vi "NIPKG to SBOM Component.vi"(8 "error in (no error)":errorcluster, 11 "nipkg package attributes":T1={"Package Name"="", "Display name"="", "Version"="", "Display version"="", "Synopsis"="", "Description"="", "Maintainer"="", "Maintainer email address"="", "Category"="", "Homepage"="", "Release notes"="", "Depends"=[], "Recommends"=[], "Suggests"=[], "Conflicts"=[], "Provides"=[], "Replaces"=[], "Supplements"=[], "Enhances"=[], "Product"=FALSE, "User visible"=FALSE, "Installed size (KB)"=0, "Package filesize (bytes)"=0, "Architecture"="", "Agent"="file", "MD5Checksum"=""}) -> (0 "error out":errorcluster, 3 "Component out":refnum<class "CycloneDX Component.lvclass">)   [LabVIEW 2017, in "NIPKG SBOM Support.lvlib"]
doc: "Converts NIPKG information to a CycloneDX SBOM component."
uses:
  NIPKG SBOM Support.lvlib
  <vilib>/National Instruments/NIPM API (Beta)/_support/package attributes.ctl
  CycloneDX/CycloneDX Component/CycloneDX Component.lvclass
  C:/LabVIEW Working Directory/labview-cyclonedx-sbom/Source/CycloneDX/CycloneDX JSON/CycloneDX JSON.lvclass
  CycloneDX/CycloneDX JSON/CycloneDX Types.ctl
  CycloneDX/CycloneDX JSON/CycloneDX JSON.lvclass
  <vilib>/National Instruments/NIPM API (Beta)/NIPM_API.lvlib
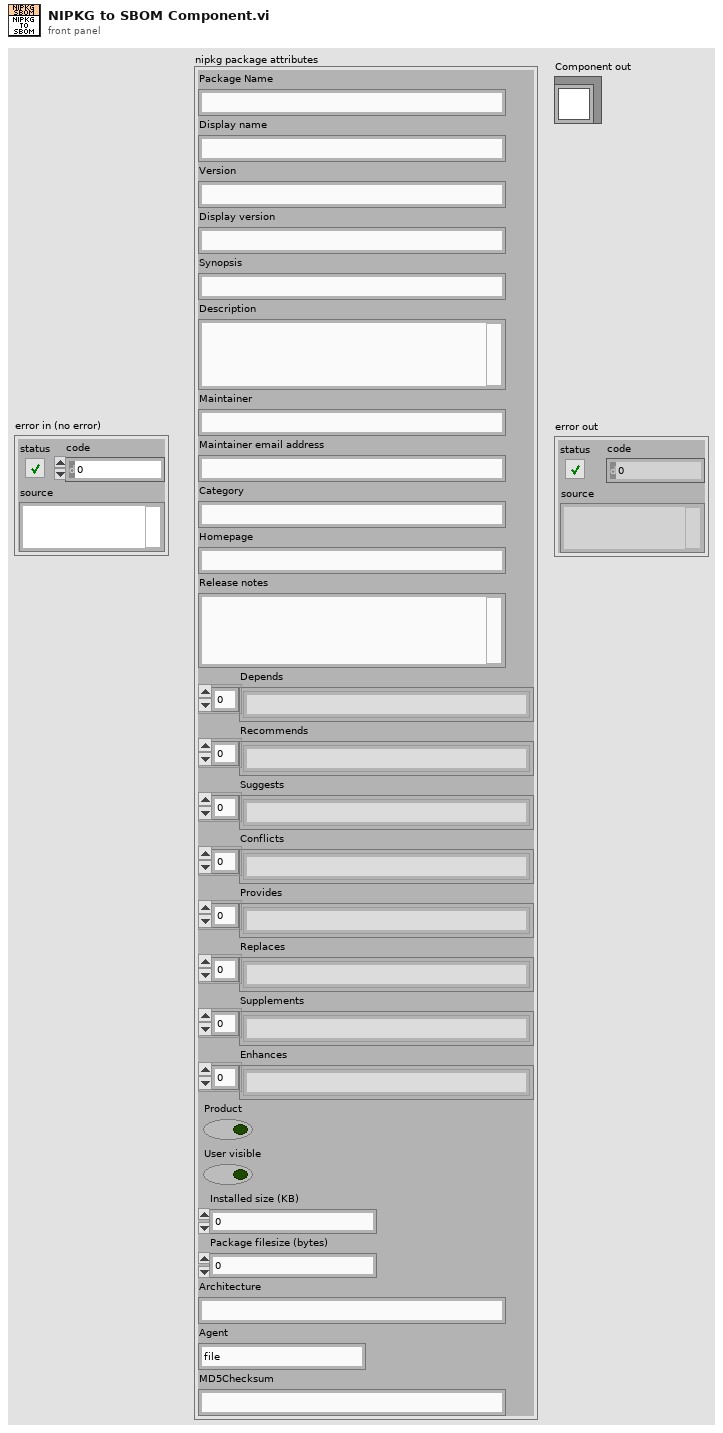
[diagram p1: front panel]
types:
  T1 = typedef "NIPM_API.lvlib/package attributes.ctl" = cluster{"Package Name":string, "Display name":string, "Version":string, "Display version":string, "Synopsis":string, "Description":string, "Maintainer":string, "Maintainer email address":string, "Category":string, "Homepage":string, "Release notes":string, "Depends":string[], "Recommends":string[], "Suggests":string[], "Conflicts":string[], "Provides":string[], "Replaces":string[], "Supplements":string[], "Enhances":string[], "Product":bool, "User visible":bool, "Installed size (KB)":u64, "Package filesize (bytes)":u64, "Architecture":string, "Agent":string, "MD5Checksum":string}
  T2 = typedef "LabVIEW CycloneDX SBOM.lvlib/CycloneDX JSON.lvclass/CycloneDX Types.ctl" = enum16{"application", "framework", "library", "container", "platform", "operating-system", "device", "device-driver", "firmware", "file", "machine-learning-model", "data"}
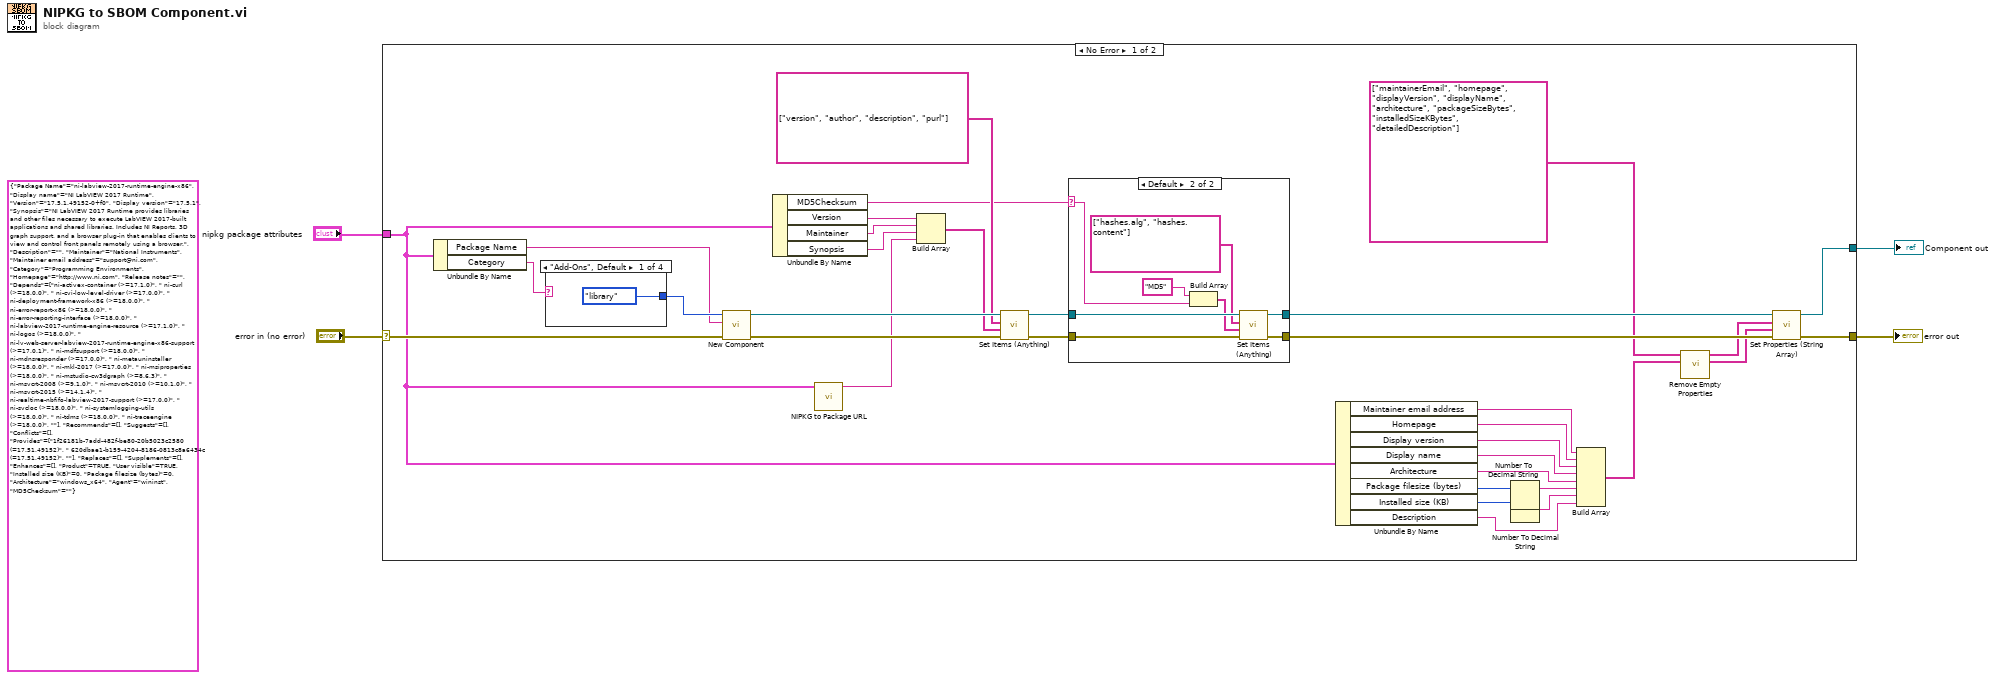
[diagram p0: block diagram]
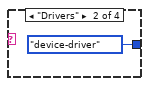
[diagram p3: hidden frame]
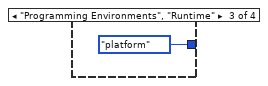
[diagram p4: hidden frame]
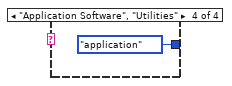
[diagram p5: hidden frame]
diagram:
  (unwired) T1 {"Package Name"="ni-labview-2017-runtime-engine-x86", "Display name"="NI LabVIEW 2017 Runtime", "Version"="17.5.1.49152-0+f0", "Display version"="17.5.1", "Synopsis"="NI LabVIEW 2017 Runtime provides libraries and other files necessary to execute LabVIEW 2017-built applications and shared libraries. Includes NI Reports, 3D graph support, and a browser plug-in that enables clients to view and control front panels remotely using a browser.", "Description"="", "Maintainer"="National Instruments", "Maintainer email address"="support@ni.com", "Category"="Programming Environments", "Homepage"="http://www.ni.com", "Release notes"="", "Depends"=["ni-activex-container (>=17.1.0)", " ni-curl (>=18.0.0)", " ni-cvi-low-level-driver (>=17.0.0)", " ni-deployment-framework-x86 (>=18.0.0)", " ni-error-report-x86 (>=18.0.0)", " ni-error-reporting-interface (>=18.0.0)", " ni-labview-2017-runtime-engine-resource (>=17.1.0)", " ni-logos (>=18.0.0)", " ni-lv-web-server-labview-2017-runtime-engine-x86-support (>=17.0.1)", " ni-mdfsupport (>=18.0.0)", " ni-mdnsresponder (>=17.0.0)", " ni-metauninstaller (>=18.0.0)", " ni-mkl-2017 (>=17.0.0)", " ni-msiproperties (>=18.0.0)", " ni-mstudio-cw3dgraph (>=8.6.3)", " ni-msvcrt-2008 (>=9.1.0)", " ni-msvcrt-2010 (>=10.1.0)", " ni-msvcrt-2015 (>=14.1.4)", " ni-realtime-nbfifo-labview-2017-support (>=17.0.0)", " ni-svcloc (>=18.0.0)", " ni-systemlogging-utils (>=18.0.0)", " ni-tdms (>=18.0.0)", " ni-traceengine (>=18.0.0)", ""], "Recommends"=[], "Suggests"=[], "Conflicts"=[], "Provides"=["1f26181b-7add-482f-be80-20b5023c2580 (=17.51.49152)", " 620dbae1-b159-4204-8186-0813c8a6434c (=17.51.49152)", ""], "Replaces"=[], "Supplements"=[], "Enhances"=[], "Product"=TRUE, "User visible"=TRUE, "Installed size (KB)"=0, "Package filesize (bytes)"=0, "Architecture"="windows_x64", "Agent"="wininst", "MD5Checksum"=""} ("package attributes")
  n1 = case shown="No Error" "error in (no error)" {
    selector: "error in (no error)" -> [w37 w53]
    tunnel: [w21 _] -> w3
    tunnel: [w20 w53] -> w2
    tunnel: "nipkg package attributes" -> [w19 _]
    frame No Error {
      n2 = Unbundle By Name(w19) -> ("Package Name"=w36:string, "Category"=w32:string)
      n3 = case shown="\"Add-Ons\", Default" w32 {
        tunnel: [CycloneDX_Types."library" ("type") CycloneDX_Types."device-driver" ("type") CycloneDX_Types."platform" ("type") CycloneDX_Types."application" ("type")] -> w38
        frame "Add-Ons", Default {
        }
        frame "Drivers" {
        }
        frame "Programming Environments", "Runtime" {
        }
        frame "Application Software", "Utilities" {
        }
      }
      n4 = call "New Component.vi"("error in (no error)"=w37, "name"=w36, "type"=w38) -> ("error out"=w35:errorcluster, "CycloneDX Component out"=w34:refnum<class "CycloneDX Component.lvclass">)  [unwired: 7 in]
      n5 = Unbundle By Name(w19) -> ("MD5Checksum"=w24:string, "Version"=w31:string, "Maintainer"=w30:string, "Synopsis"=w29:string)
      n6 = call "NIPKG to Package URL.vi"("package attributes"=w19) -> ("NIPKG Package URL"=w28:string)  [unwired: 10 in]
      n7 = Build Array(w31, w30, w29, w28) -> (w27:string[])
      n8 = call "Set Items (Anything).vi"("error in (no error)"=w35, "Value"=w27, "Item Paths"=string[] ["version", "author", "description", "purl"], "CycloneDX SBOM in"=w34) -> ("error out"=w26:errorcluster, "CycloneDX SBOM out"=w25:refnum<class "CycloneDX Component.lvclass">)  [unwired: 6 in]
      n9 = case shown="Default" w24 {
        selector: w24 -> [_ w43]
        tunnel: w26 -> [w39 w48]
        tunnel: [w39 w47] -> w23
        tunnel: w25 -> [w40 w46]
        tunnel: [w40 w45] -> w22
        frame "" {
        }
        frame Default {
          n10 = Build Array("MD5", w43) -> (w41:string[])
          n11 = call "Set Items (Anything).vi"("error in (no error)"=w48, "Value"=w41, "Item Paths"=string[] ["hashes.alg", "hashes.content"], "CycloneDX SBOM in"=w46) -> ("error out"=w47:errorcluster, "CycloneDX SBOM out"=w45:refnum<class "CycloneDX Component.lvclass">)  [unwired: 6 in]
        }
      }
      n12 = Unbundle By Name(w19) -> ("Maintainer email address"=w18:string, "Homepage"=w17:string, "Display version"=w16:string, "Display name"=w15:string, "Architecture"=w14:string, "Package filesize (bytes)"=w13:u64, "Installed size (KB)"=w11:u64, "Description"=w9:string)
      n13 = Number To Decimal String(number=w13) -> (decimal integer string=w12:string)  [unwired: 1 in]
      n14 = Number To Decimal String(number=w11) -> (decimal integer string=w10:string)  [unwired: 1 in]
      n15 = Build Array(w18, w17, w16, w15, w14, w12, w10, w9) -> (w8:string[])
      n16 = call "Remove Empty Properties.vi"("Values in"=w8, "Names in"=string[] ["maintainerEmail", "homepage", "displayVersion", "displayName", "architecture", "packageSizeBytes", "installedSizeKBytes", "detailedDescription"]) -> ("Values out"=w5:string[], "Names out"=w6:string[])  [unwired: 8 in]
      n17 = call "Set Properties (String Array).vi"("error in (no error)"=w23, "values (string)"=w5, "names"=w6, "CycloneDX JSON in"=w22) -> ("error out"=w20:errorcluster, "CycloneDX JSON out"=w21:refnum<class "CycloneDX Component.lvclass">)  [unwired: 6 in]
    }
    frame Error {
    }
  }
  "error out" <- w2
  "Component out" <- w3
